vi "Add Menu Item.vi"(8 "error in (no error)":errorcluster, 10 "Item Names":string[](array[string]), 11 "Queed Listbox ref":refnum<vi>) -> (0 "error out":errorcluster, 2 "Current Strings":string[](array[string]), 3 "Queed Listbox ref out":refnum<vi>)   [LabVIEW 2015]
uses:
  Queued Listbox.xctl
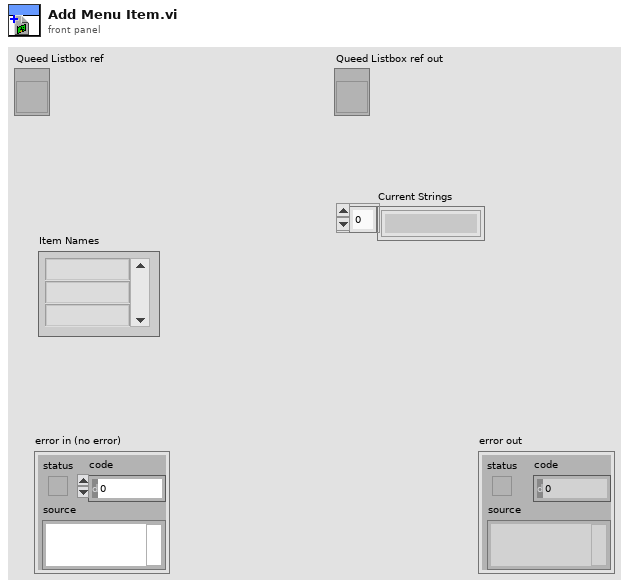
[diagram p1: front panel]
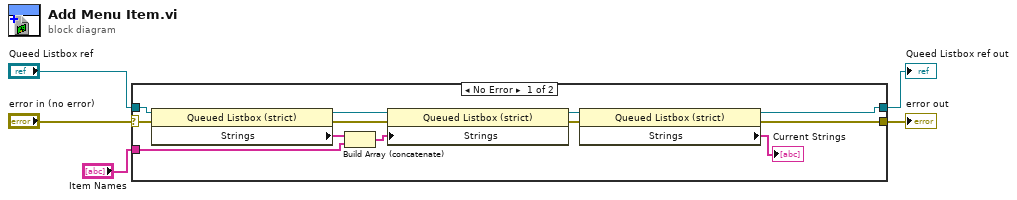
[diagram p0: block diagram]
diagram:
  n1 = case shown="No Error" "error in (no error)" {
    selector: "error in (no error)" -> [w14 w19]
    tunnel: [w9 w19] -> w3
    tunnel: "Item Names" -> [w15 _]
    tunnel: "Queed Listbox ref" -> [w7 w18]
    tunnel: [w6 w18] -> w1
    frame No Error {
      n2 = property class="Queued Listbox (strict)"(reference=w7, error in=w14) -> (reference out=w17:refnum<vi>, error out=w13:errorcluster, "Strings"=w16:string[])
      n3 = Build Array (concatenate)(w16, w15) -> (w12:string[])
      n4 = property class="Queued Listbox (strict)"(reference=w17, error in=w13, "Strings"=w12) -> (reference out=w10:refnum<vi>, error out=w11:errorcluster)
      n5 = property class="Queued Listbox (strict)"(reference=w10, error in=w11) -> (reference out=w6:refnum<vi>, error out=w9:errorcluster, "Strings"=→"Current Strings":string[])
    }
    frame Error {
    }
  }
  "error out" <- w3
  "Queed Listbox ref out" <- w1
